vi "dés.vi"() -> ()   [LabVIEW 2018]
panel:
  out "led 1":bool
  out "led7":bool
  out "led 5":bool
  out "led 2":bool
  out "led 4":bool
  out "led 6":bool
  out "led 3":bool
  in  "Numeric":u32=1 min=1 max=7
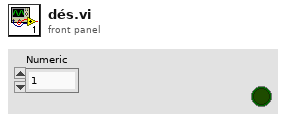
[diagram p1: front panel]
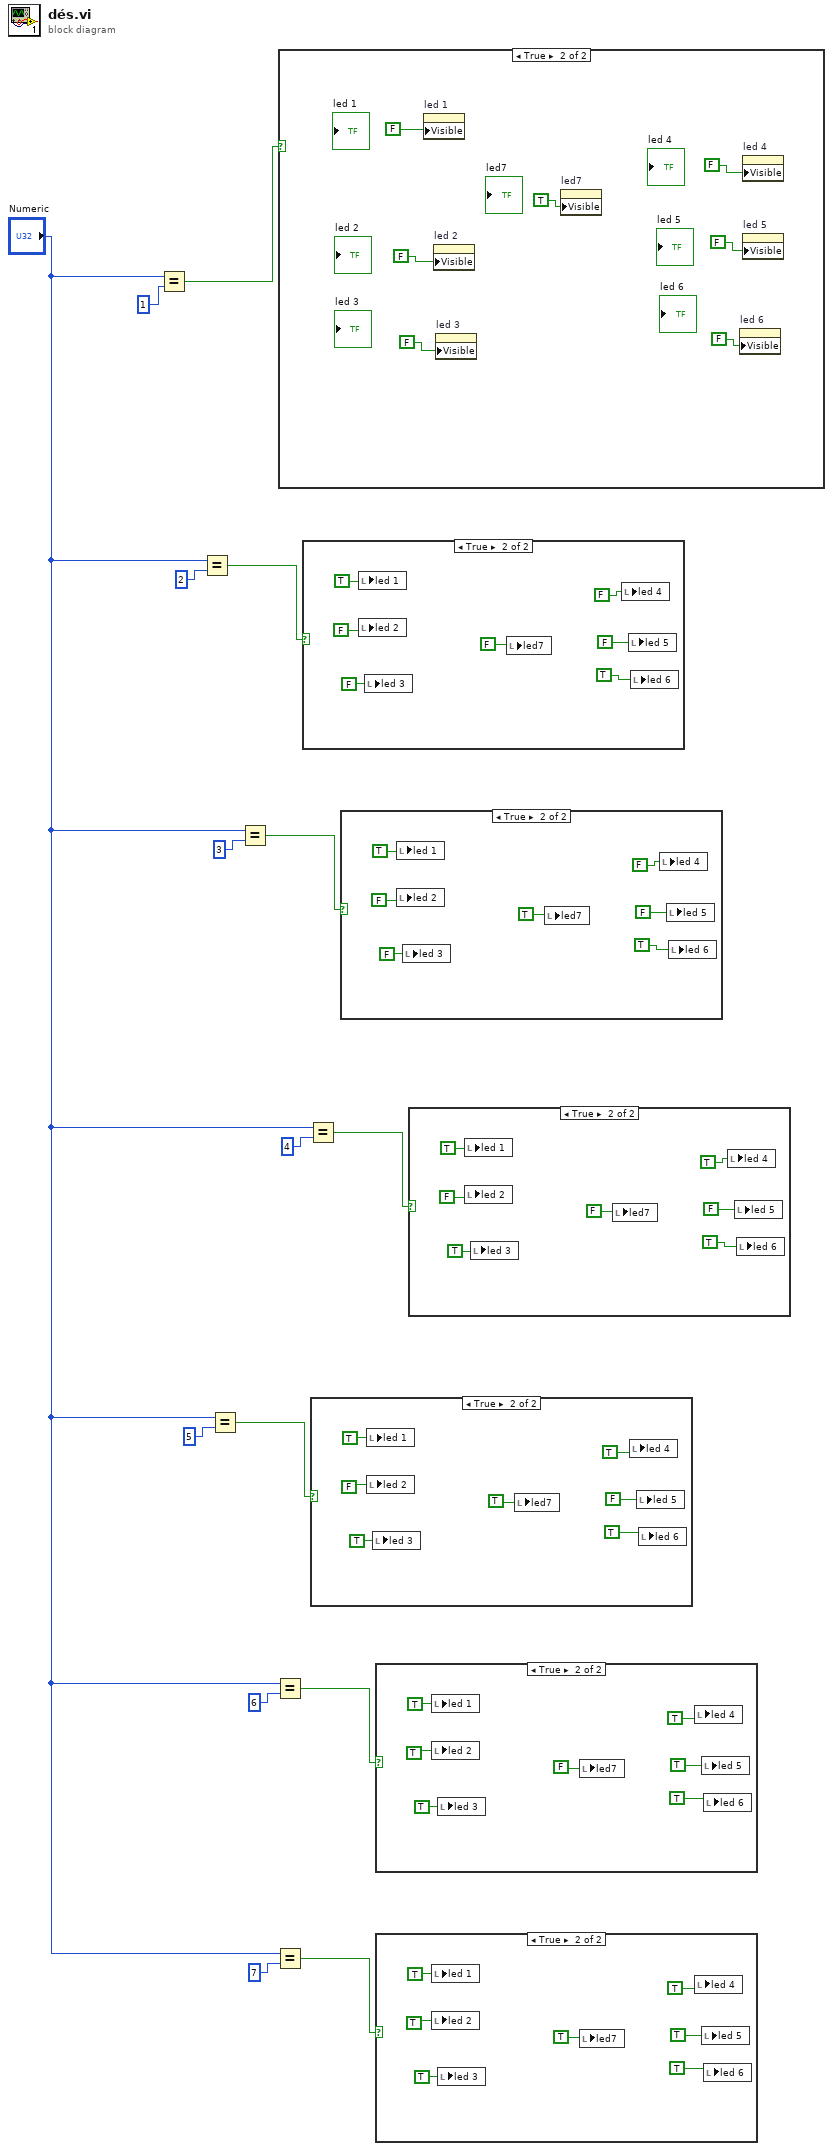
[diagram p0: block diagram]
diagram:
  n1 = Equal?(x="Numeric", y=1) -> (x = y?=w14:bool)
  n2 = Equal?(x="Numeric", y=2) -> (x = y?=w12:bool)
  n3 = Equal?(x="Numeric", y=5) -> (x = y?=w6:bool)
  n4 = Equal?(x="Numeric", y=3) -> (x = y?=w8:bool)
  n5 = Equal?(x="Numeric", y=6) -> (x = y?=w4:bool)
  n6 = Equal?(x="Numeric", y=7) -> (x = y?=w2:bool)
  n7 = case shown="True" w14 {
    frame False {
    }
    frame True {
      n8 = property on="led 1" class="Bool (strict)"("Visible"=FALSE) -> ()  [unwired: 2 in, 2 out]
      n9 = property on="led 2" class="Bool (strict)"("Visible"=FALSE) -> ()  [unwired: 2 in, 2 out]
      n10 = property on="led 3" class="Bool (strict)"("Visible"=FALSE) -> ()  [unwired: 2 in, 2 out]
      n11 = property on="led7" class="Bool (strict)"("Visible"=TRUE) -> ()  [unwired: 2 in, 2 out]
      n12 = property on="led 6" class="Bool (strict)"("Visible"=FALSE) -> ()  [unwired: 2 in, 2 out]
      n13 = property on="led 4" class="Bool (strict)"("Visible"=FALSE) -> ()  [unwired: 2 in, 2 out]
      n14 = property on="led 5" class="Bool (strict)"("Visible"=FALSE) -> ()  [unwired: 2 in, 2 out]
    }
  }
  n15 = case shown="True" w12 {
    frame False {
    }
    frame True {
      n16 = local write "led 1"(TRUE) -> ()
      n17 = local write "led 2"(FALSE) -> ()
      n18 = local write "led 3"(FALSE) -> ()
      n19 = local write "led7"(FALSE) -> ()
      n20 = local write "led 4"(FALSE) -> ()
      n21 = local write "led 5"(FALSE) -> ()
      n22 = local write "led 6"(TRUE) -> ()
    }
  }
  n23 = Equal?(x="Numeric", y=4) -> (x = y?=w10:bool)
  n24 = case shown="True" w6 {
    frame False {
    }
    frame True {
      n25 = local write "led 1"(TRUE) -> ()
      n26 = local write "led 2"(FALSE) -> ()
      n27 = local write "led 3"(TRUE) -> ()
      n28 = local write "led7"(TRUE) -> ()
      n29 = local write "led 4"(TRUE) -> ()
      n30 = local write "led 5"(FALSE) -> ()
      n31 = local write "led 6"(TRUE) -> ()
    }
  }
  n32 = case shown="True" w8 {
    frame False {
    }
    frame True {
      n33 = local write "led 1"(TRUE) -> ()
      n34 = local write "led 2"(FALSE) -> ()
      n35 = local write "led 3"(FALSE) -> ()
      n36 = local write "led7"(TRUE) -> ()
      n37 = local write "led 4"(FALSE) -> ()
      n38 = local write "led 5"(FALSE) -> ()
      n39 = local write "led 6"(TRUE) -> ()
    }
  }
  n40 = case shown="True" w4 {
    frame False {
    }
    frame True {
      n41 = local write "led 1"(TRUE) -> ()
      n42 = local write "led 2"(TRUE) -> ()
      n43 = local write "led 3"(TRUE) -> ()
      n44 = local write "led7"(FALSE) -> ()
      n45 = local write "led 4"(TRUE) -> ()
      n46 = local write "led 5"(TRUE) -> ()
      n47 = local write "led 6"(TRUE) -> ()
    }
  }
  n48 = case shown="True" w2 {
    frame False {
    }
    frame True {
      n49 = local write "led 1"(TRUE) -> ()
      n50 = local write "led 2"(TRUE) -> ()
      n51 = local write "led 3"(TRUE) -> ()
      n52 = local write "led7"(TRUE) -> ()
      n53 = local write "led 4"(TRUE) -> ()
      n54 = local write "led 5"(TRUE) -> ()
      n55 = local write "led 6"(TRUE) -> ()
    }
  }
  n56 = case shown="True" w10 {
    frame False {
    }
    frame True {
      n57 = local write "led 1"(TRUE) -> ()
      n58 = local write "led 2"(FALSE) -> ()
      n59 = local write "led 3"(TRUE) -> ()
      n60 = local write "led7"(FALSE) -> ()
      n61 = local write "led 4"(TRUE) -> ()
      n62 = local write "led 5"(FALSE) -> ()
      n63 = local write "led 6"(TRUE) -> ()
    }
  }
